vi "number1_sub1-login.vi"() -> (1 "UserCancelled":bool, 2 "Correct":bool)   [LabVIEW 2014]
panel:
  in  "Cancel":bool
  in  "Login":bool
  in  "Password":string
  in  "Username":string
  # "(user)"
  # "(password)"
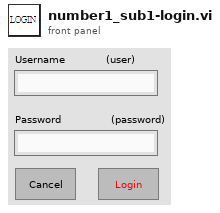
[diagram p1: front panel]
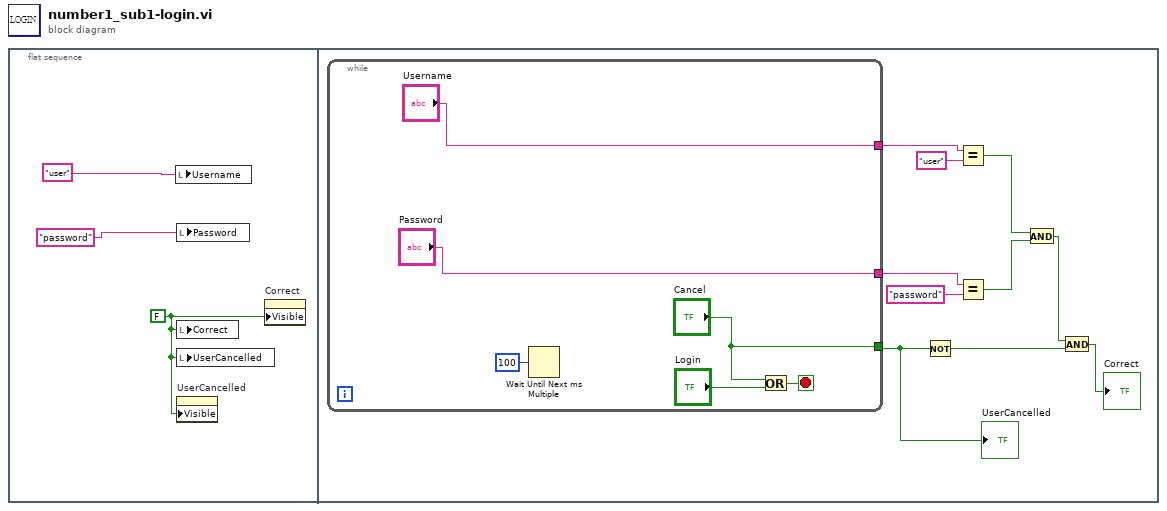
[diagram p0: block diagram]
diagram:
  n1 = flat-sequence {
    frame #0 {
      w3 = FALSE ("Correct")
      n2 = local write "Username"("user" ("Username")) -> ()
      n3 = local write "Password"("password" ("Password")) -> ()
      n4 = local write "Correct"(w3) -> ()
      n5 = local write "UserCancelled"(w3) -> ()
      n6 = property on="UserCancelled" class="Bool (strict)"("Visible"=w3) -> ()  [unwired: 2 in, 2 out]
      n7 = property on="Correct" class="Bool (strict)"("Visible"=w3) -> ()  [unwired: 2 in, 2 out]
    }
    frame #1 {
      n8 = while {
        tunnel: ["Username"] -> w9
        tunnel: ["Password"] -> w8
        tunnel: ["Cancel"] -> w4
        stop <- w16 stop-if-true
        n9 = Wait Until Next ms Multiple(millisecond multiple=u32 100) -> ()  [unwired: 1 out]
        n10 = Or(x="Cancel", y="Login") -> (x .or. y?=w16:bool)
      }
      "UserCancelled" <- w4
      n11 = Not(x=w4) -> (.not. x?=w6:bool)
      n12 = Equal?(x=w9, y="user") -> (x = y?=w12:bool)
      n13 = Equal?(x=w8, y="password") -> (x = y?=w13:bool)
      n14 = And(x=w12, y=w13) -> (x .and. y?=w5:bool)
      n15 = And(x=w5, y=w6) -> (x .and. y?=→"Correct":bool)
    }
  }
